vi "(Sub_VI)_Randomize_ArrayofCluster.vi"(2 "Orig Array":dbl[][](array[numeric]), 3 "Randomize or not":bool) -> (0 "Randomized Index":i32[](array[numeric]), 1 "Randomized Array in 2nd Dimension":dbl[][](array[numeric]))   [LabVIEW 2012]
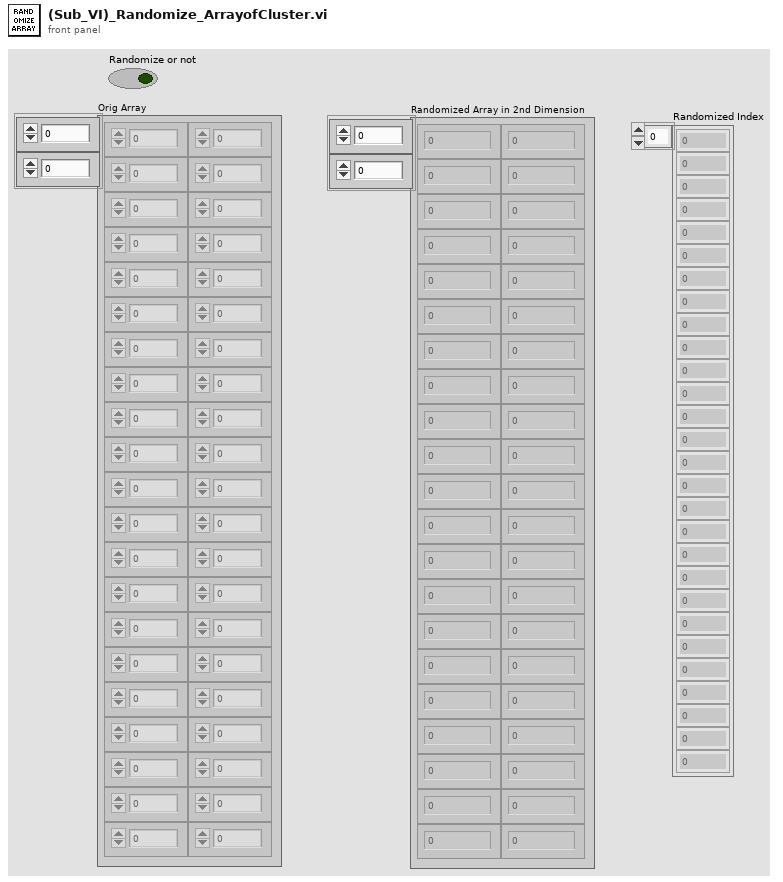
[diagram p1: front panel]
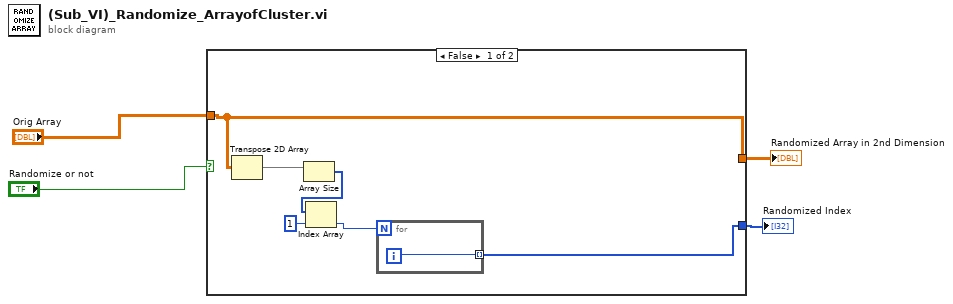
[diagram p0: block diagram]
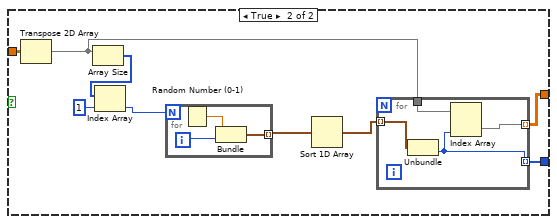
[diagram p2: hidden frame]
diagram:
  n1 = case shown="False" "Randomize or not" {
    tunnel: "Orig Array" -> [w6 w18]
    tunnel: [w5 w14] -> w3
    tunnel: [w6 w12] -> w2
    frame False {
      n2 = Transpose 2D Array(2D array=w6) -> (transposed array=w7:dbl[][])
      n3 = Array Size(array=w7) -> (size(s)=w10:i32[])
      n4 = Index Array(array=w10, index=1) -> (element=w8:i32)
      n5 = for {
        N: w8 -> [_]
        tunnel: [w11] -> w5 mode=indexing
        i -> [w11]
      }
    }
    frame True {
      n6 = Transpose 2D Array(2D array=w18) -> (transposed array=w13:dbl[][])
      n7 = Array Size(array=w13) -> (size(s)=w17:i32[])
      n8 = Index Array(array=w17, index=1) -> (element=w15:i32)
      n9 = for {
        N: w15 -> [_]
        tunnel: [w25] -> w20 mode=indexing
        i -> [w26]
        n10 = Random Number (0-1)() -> (number: 0 to 1=w27:dbl)
        n11 = Bundle("number: 0 to 1"=w27, w26) -> (w25:cluster{"number: 0 to 1":dbl, i32})  [unwired: 1 in]
      }
      n12 = Sort 1D Array(array=w20) -> (sorted array=w19:cluster{"number: 0 to 1":dbl, i32}[])
      n13 = for {
        tunnel: w19 -> [w24] mode=indexing
        tunnel: w13 -> [w23]
        tunnel: [w22] -> w12 mode=indexing
        tunnel: [w21] -> w14 mode=indexing
        n14 = Unbundle(w24) -> (w21:i32)  [unwired: 1 out]
        n15 = Index Array(array=w23, index (col)=w21) -> (element=w22:dbl[])  [unwired: 1 in]
      }
    }
  }
  "Randomized Array in 2nd Dimension" <- w2
  "Randomized Index" <- w3
